vi "OneMonthLaterSubVI.vi"(0 "timestamp":timestamp) -> (1 "current date":string, 2 "one month later date":string)   [LabVIEW 2011]
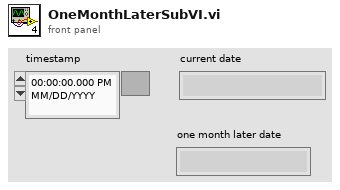
[diagram p1: front panel]
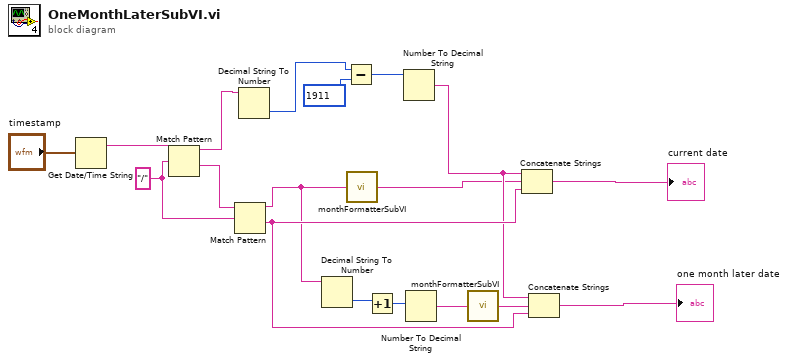
[diagram p0: block diagram]
diagram:
  w4 = "/" ("search string/char (-)")
  n1 = Get Date/Time String(seconds (now)="timestamp") -> (date string=w2:string)  [unwired: 2 in, 1 out]
  n2 = Match Pattern(string=w2, regular expression=w4) -> (before substring=w5:string, after substring=w3:string)  [unwired: 1 in, 2 out]
  n3 = Match Pattern(string=w3, regular expression=w4) -> (before substring=w12:string, after substring=w17:string)  [unwired: 1 in, 2 out]
  n4 = Decimal String To Number(string=w5) -> (number=w6:i32)  [unwired: 2 in, 1 out]
  n5 = Decimal String To Number(string=w12) -> (number=w10:i32)  [unwired: 2 in, 1 out]
  n6 = Subtract(x=w6, y=1911) -> (x-y=w8:i32)
  n7 = call "monthFormatterSubVI.vi"("month string in"=w12) -> ("month string out"=w13:string)
  n8 = Increment(x=w10) -> (x+1=w11:i32)
  n9 = Number To Decimal String(number=w8) -> (decimal integer string=w16:string)  [unwired: 1 in]
  n10 = Number To Decimal String(number=w11) -> (decimal integer string=w14:string)  [unwired: 1 in]
  n11 = call "monthFormatterSubVI.vi"("month string in"=w14) -> ("month string out"=w15:string)
  n12 = Concatenate Strings(w16, w13, w17) -> (→"current date":string)
  n13 = Concatenate Strings(w16, w15, w17) -> (→"one month later date":string)
